vi "FreqtoTicks.vi"(2 "Boolean":bool, 3 "Frequency":dbl) -> (0 "Boolean 2":bool, 1 "Numeric":u32)   [LabVIEW 8.6]
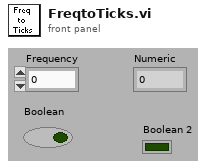
[diagram p1: front panel]
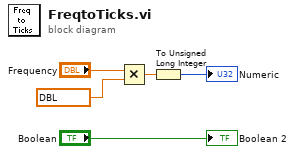
[diagram p0: block diagram]
diagram:
  n1 = Multiply(x="Frequency", y=dbl ?) -> (x*y=w4:dbl)
  n2 = To Unsigned Long Integer(number=w4) -> (unsigned 32bit integer=→"Numeric":u32)
  "Boolean 2" <- "Boolean"
